vi "PV Software Extract HEX Data.vi"(8 "error in (no error)":errorcluster, 11 "All Data":string[][](array[string])) -> (0 "error out":errorcluster, 2 "Date and Time":string[][](array[string]), 3 "HEX Data (String)":string[](array[string]))   [LabVIEW 2023]
uses:
  <vilib>/Utility/error.llb/whitespace.ctl
  <vilib>/Utility/error.llb/Trim Whitespace One-Sided.vi
panel:
  out "Array 3":string[](array[string])
  # "Test Mode 1 = 6 Bytes\nTest Mode 2 = 8 Bytes\nVOC Sensor = 3 Bytes\nDHW = 2 Bytes"
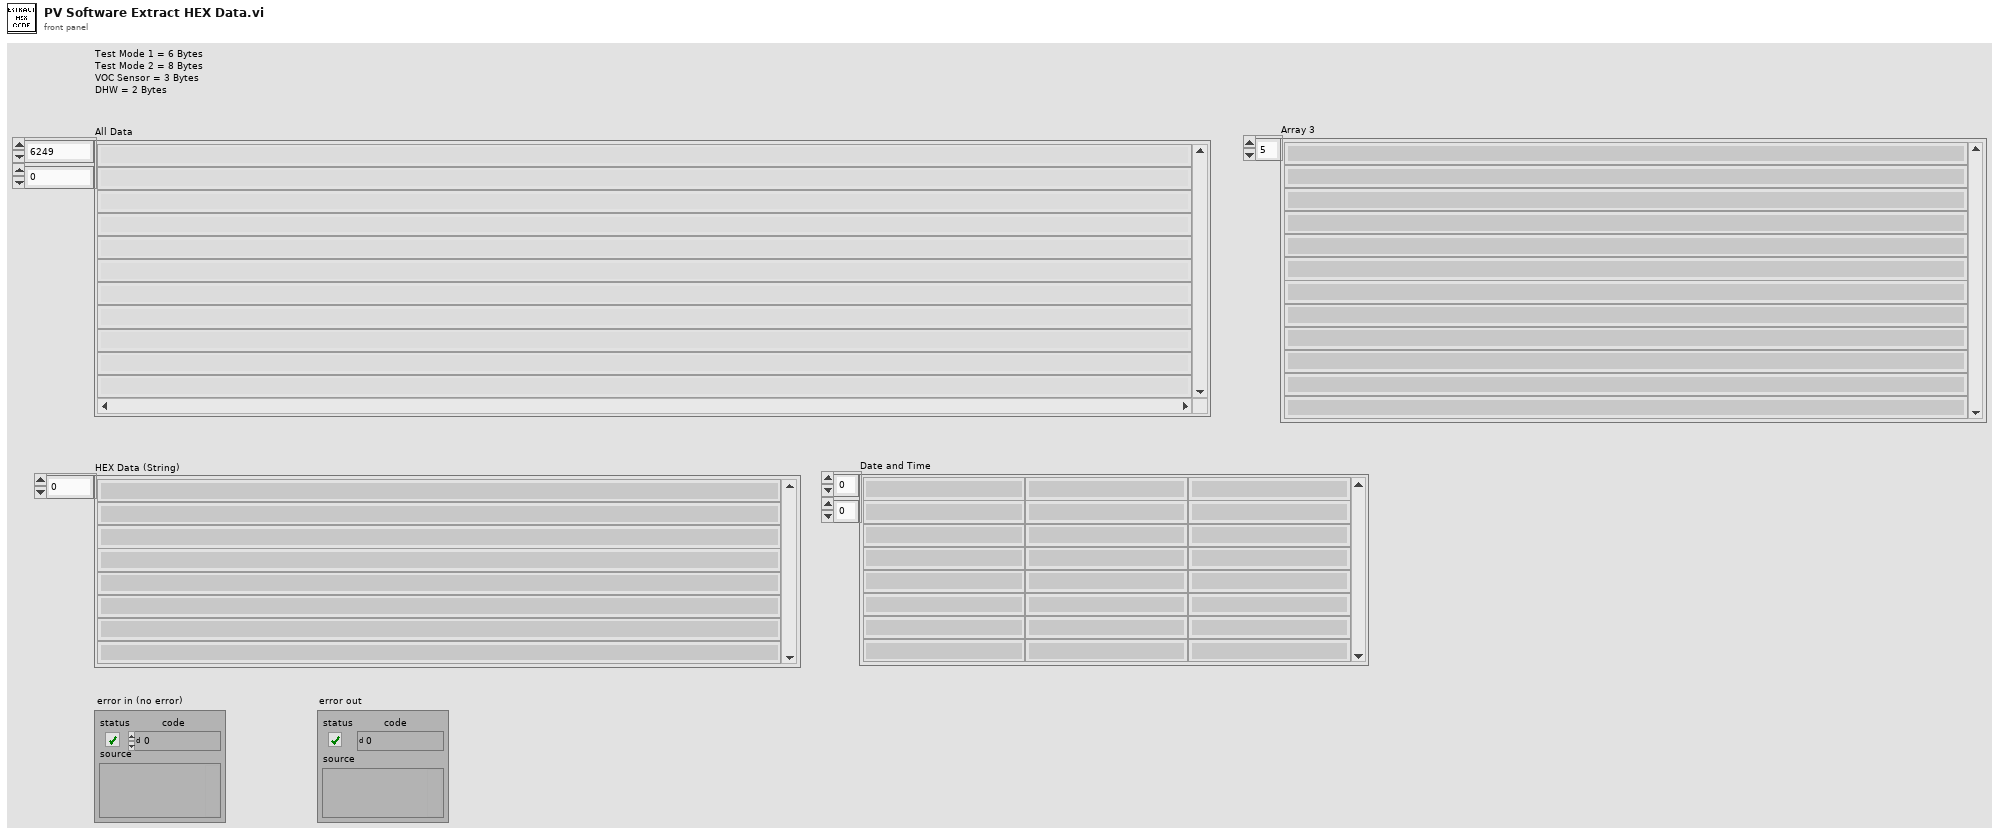
[diagram p1: front panel]
types:
  T1 = typedef "whitespace.ctl" = u16
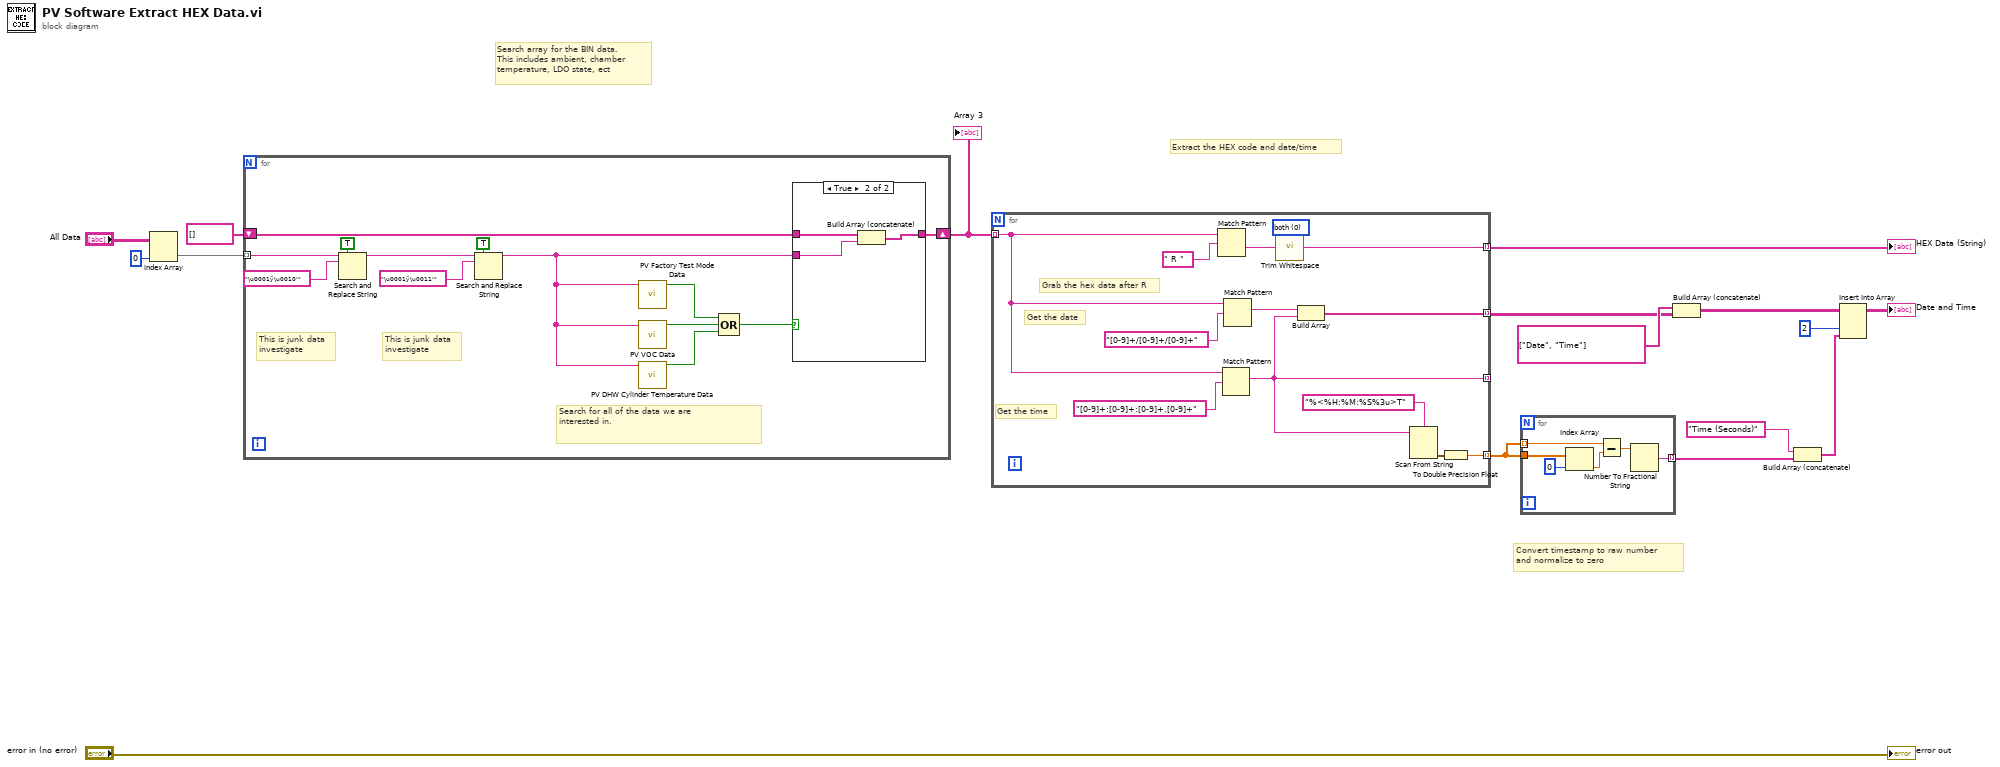
[diagram p0: block diagram]
diagram:
  # "Convert timestamp to raw number \nand normalize to zero"
  # "Extract the HEX code and date/time"
  # "Search array for the BIN data. \nThis includes ambient, chamber \ntemperature, LDO state, ect"
  n1 = Index Array(array="All Data", index (col)=0 ("disabled index (col)")) -> (element=w13:string[])  [unwired: 1 in]
  n2 = for {
    tunnel: w13 -> [w25] mode=indexing
    shift-right: [w28] -> w15
    shift-left: string[] [] -> [w29]
    # "Search for all of the data we are \ninterested in."
    # "This is junk data\ninvestigate"
    # "This is junk data\ninvestigate"
    n3 = Search and Replace String(replace all?=TRUE ("replace all? (F)"), input string=w25, search string="\u0001ÿ\u0010'") -> (result string=w22:string)  [unwired: 5 in, 3 out]
    n4 = Search and Replace String(replace all?=TRUE ("replace all? (F)"), input string=w22, search string="\u0001ÿ\u0011'") -> (result string=w21:string)  [unwired: 5 in, 3 out]
    n5 = call "PV Factory Test Mode Data.vi"("result string"=w21) -> ("Boolean"=w20:bool)  [unwired: 10 in]
    n6 = call "PV VOC Data.vi"("result string"=w21) -> ("Boolean"=w19:bool)  [unwired: 10 in]
    n7 = call "PV DHW Cylinder Temperature Data.vi"("result string"=w21) -> ("Boolean"=w18:bool)  [unwired: 10 in]
    n8 = Compound Arithmetic op=OR(w20, w19, w18) -> (w17:bool)
    n9 = case shown="True" w17 {
      tunnel: w29 -> [w30 w33]
      tunnel: [w30 w32] -> w28
      tunnel: w21 -> [_ w31]
      frame False {
      }
      frame True {
        n10 = Build Array (concatenate)(w33, w31) -> (w32:string[])
      }
    }
  }
  "Array 3" <- w15
  n11 = for {
    tunnel: w15 -> [w40] mode=indexing
    tunnel: [w43] -> w16 mode=indexing
    tunnel: [w38] -> w8 mode=indexing
    tunnel: [w35] -> _ mode=indexing
    tunnel: [w34] -> w7 mode=indexing
    w45 = T1 0 items=["both", "start of string", "end of string"] ("location (both)")
    # "Get the time"
    # "Get the date"
    # "Grab the hex data after R"
    n12 = Match Pattern(string=w40, regular expression=" R " ("string")) -> (after substring=w44:string)  [unwired: 1 in, 3 out]
    n13 = Match Pattern(string=w40, regular expression="[0-9]+:[0-9]+:[0-9]+.[0-9]+" ("string")) -> (match substring=w35:string)  [unwired: 1 in, 3 out]
    n14 = Match Pattern(string=w40, regular expression="[0-9]+/[0-9]+/[0-9]+" ("string")) -> (match substring=w39:string)  [unwired: 1 in, 3 out]
    n15 = call <vilib>:"Trim Whitespace.vi"("string"=w44, "location (both)"=w45) -> ("trimmed string"=w43:string)
    n16 = Build Array(w39, w35) -> (w38:string[])
    n17 = Scan From String(format string="%<%H:%M:%S%3u>T", input string=w35) -> (output 1=w37:timestamp)  [unwired: 3 in, 3 out]
    n18 = To Double Precision Float(number=w37) -> (double precision float=w34:dbl)
  }
  "HEX Data (String)" <- w16
  n19 = for {
    tunnel: w7 -> [w52]
    tunnel: w7 -> [w50] mode=indexing
    tunnel: [w47] -> w5 mode=indexing
    n20 = Index Array(array=w52, index=0) -> (element=w49:dbl)
    n21 = Subtract(x=w50, y=w49) -> (x-y=w48:dbl)
    n22 = Number To Fractional String(number=w48) -> (F-format string=w47:string)  [unwired: 3 in]
  }
  n23 = Build Array (concatenate)(string[] ["Date", "Time"], w8) -> (w4:string[][])
  n24 = Build Array (concatenate)("Time (Seconds)", w5) -> (w3:string[])
  n25 = Insert Into Array(array=w4, index (col)=2 ("disabled index (col)"), new element=w3) -> (→"Date and Time":string[][])  [unwired: 1 in]
  "error out" <- "error in (no error)"
